vi "Convert TimeStamp To Double.vi"() -> ()   [LabVIEW 2014]
panel:
  out "Numeric":dbl
  in  "Time Stamp":timestamp format="%<%H:%M:%S%4u\n%x>T"
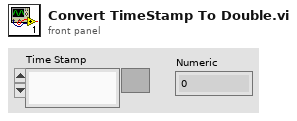
[diagram p1: front panel]
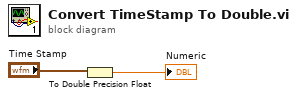
[diagram p0: block diagram]
diagram:
  n1 = To Double Precision Float(number="Time Stamp") -> (double precision float=→"Numeric":dbl)
